vi "SpikeTimingCount_003.vi"(1 "template":i32[](array[numeric]), 2 "Test object":i32[](array[numeric]), 3 "Total Duration":i32, 4 "Number of Bins":i32) -> (0 "Dissimilarity":dbl)   [LabVIEW 2018]
panel:
  out "Test Check":dbl[](array[numeric])
  out "Template Check":dbl[](array[numeric])
  out "x .xor. y?":bool[](array[boolean])
  out "Template":bool[](array[boolean])
  out "Test Object":bool[](array[boolean])
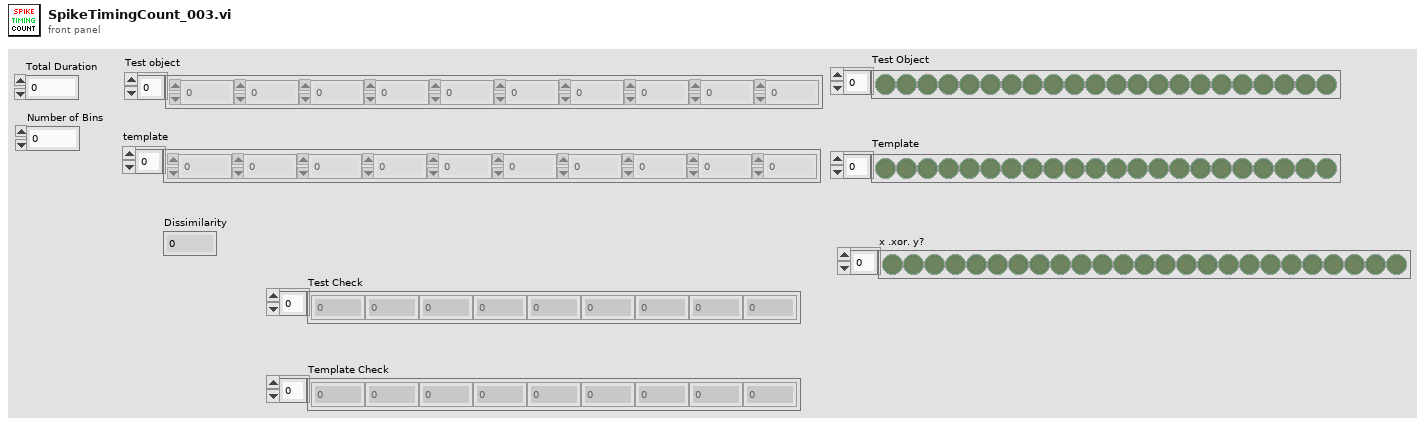
[diagram p1: front panel]
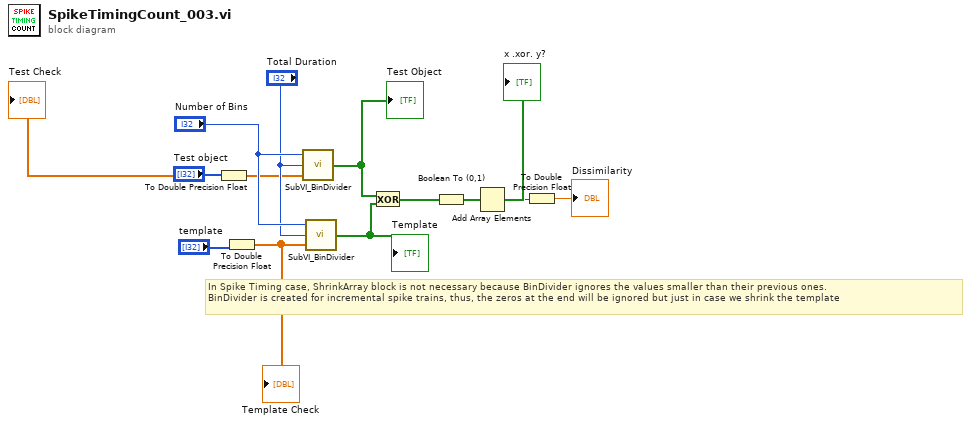
[diagram p0: block diagram]
diagram:
  # "In Spike Timing case, ShrinkArray block is not necessary because BinDivider ignores the values smaller than their previous ones.\nBinDivider is created for incremental spike trains, thus, the zeros at the end will be ignored but just in case we shrink the template"
  n1 = To Double Precision Float(number="Test object") -> (double precision float=w2:dbl[])
  "Test Check" <- w2
  n2 = To Double Precision Float(number="template") -> (double precision float=w4:dbl[])
  "Template Check" <- w4
  n3 = call "SubVI_BinDivider.vi"("Spike Times"=w2, "Total Duration [ms]"="Total Duration", "Number of Bins"="Number of Bins") -> ("Array"=w7:bool[])
  "Test Object" <- w7
  n4 = call "SubVI_BinDivider.vi"("Spike Times"=w4, "Total Duration [ms]"="Total Duration", "Number of Bins"="Number of Bins") -> ("Array"=w12:bool[])
  "Template" <- w12
  n5 = Exclusive Or(1:w12, 2:w7) -> (0:w11:bool[])
  "x .xor. y?" <- w11
  n6 = Boolean To (0,1)(Boolean=w11) -> (0, 1=w10:i16[])
  n7 = Add Array Elements(numeric array=w10) -> (sum=w6:i16)
  n8 = To Double Precision Float(number=w6) -> (double precision float=→"Dissimilarity":dbl)
